vi "SUB_OUT_THIS_token.vi"(2 "Remove token symbl1 3":string, 3 "Remove token symbl1 2":string, 4 "Remove token symbl1":string, 5 "input string":string) -> (1 "result string":string)   [LabVIEW 2011]
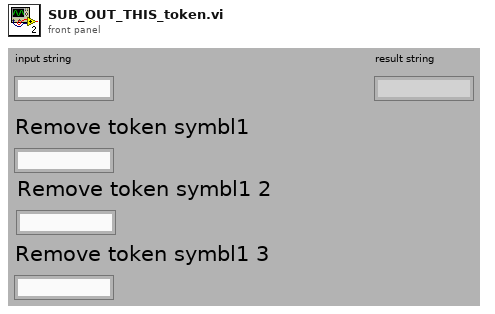
[diagram p1: front panel]
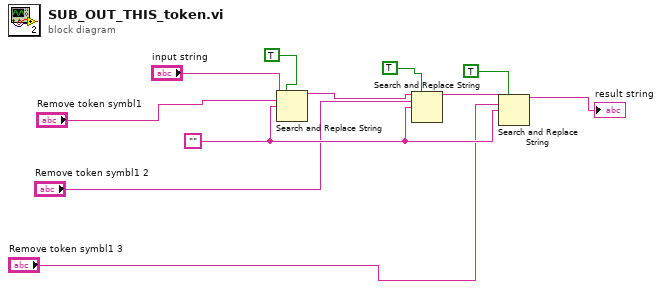
[diagram p0: block diagram]
diagram:
  w6 = ""
  n1 = Search and Replace String(replace all?=TRUE ("replace all? (F)"), input string="input string", search string="Remove token symbl1", replace string=w6) -> (result string=w11:string)  [unwired: 4 in, 3 out]
  n2 = Search and Replace String(replace all?=TRUE ("ignore case? (F)"), input string=w11, search string="Remove token symbl1 2", replace string=w6) -> (result string=w7:string)  [unwired: 4 in, 3 out]
  n3 = Search and Replace String(replace all?=TRUE ("replace all? (F)"), input string=w7, search string="Remove token symbl1 3", replace string=w6) -> (result string=→"result string":string)  [unwired: 4 in, 3 out]
